vi "Linear Spacing.vi"() -> ()   [LabVIEW 2015]
panel:
  in  "Enum":enum16{"Linear", "Logrithmic"}(ring)
  out "Waveform Graph":dbl[](graph)
  out "Linear":dbl[](array[numeric])
  in  "Number of Elements":i32
  in  "Min":dbl
  in  "Max":dbl
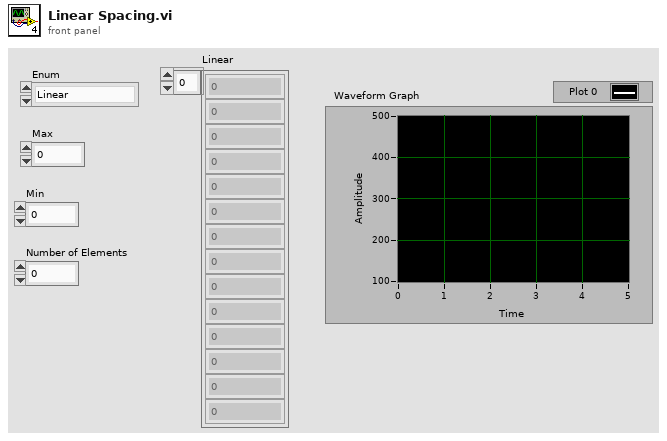
[diagram p1: front panel]
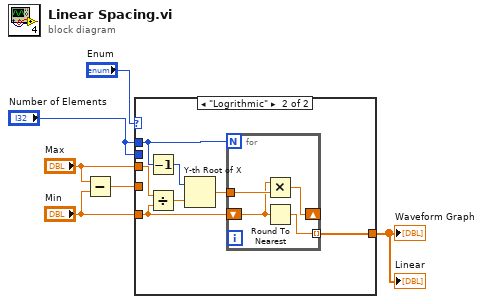
[diagram p0: block diagram]
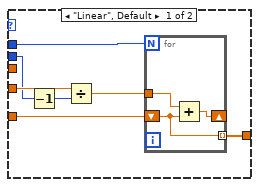
[diagram p2: hidden frame]
diagram:
  n1 = Subtract(x="Max", y="Min") -> (x-y=w6:dbl)
  n2 = case shown="\"Logrithmic\"" "Enum" {
    tunnel: w6 -> [w12 _]
    tunnel: "Min" -> [w11 w18]
    tunnel: [w10 w21] -> w4
    tunnel: "Number of Elements" -> [w9 w20]
    tunnel: "Max" -> [_ w19]
    tunnel: "Number of Elements" -> [w8 _]
    frame "Linear", Default {
      n3 = Decrement(x=w8) -> (x-1=w7:i32)
      n4 = Divide(x=w12, y=w7) -> (x/y=w13:dbl)
      n5 = for {
        N: w9 -> [_]
        tunnel: w13 -> [w16]
        tunnel: [w15] -> w10 mode=indexing
        shift-right: [w14] -> _
        shift-left: w11 -> [w15]
        n6 = Add(x=w16, y=w15) -> (x+y=w14:dbl)
      }
    }
    frame "Logrithmic" {
      n7 = Decrement(x=w20) -> (x-1=w17:i32)
      n8 = Divide(x=w19, y=w18) -> (x/y=w22:dbl)
      n9 = Y-th Root of X(1:w22, 2:w17) -> (0:w23:dbl)
      n10 = for {
        N: w20 -> [_]
        tunnel: w23 -> [w27]
        tunnel: [w24] -> w21 mode=indexing
        shift-right: [w26] -> _
        shift-left: w18 -> [w25]
        n11 = Multiply(x=w25, y=w27) -> (x*y=w26:dbl)
        n12 = Round To Nearest(number=w25) -> (nearest integer value=w24:dbl)
      }
    }
  }
  "Linear" <- w4
  "Waveform Graph" <- w4
